vi "Close File.vi"(8 "error in (no error)":errorcluster, 11 "Macro in":refnum<class "Macro.lvclass">) -> (0 "error out":errorcluster, 3 "Macro out":refnum<class "Macro.lvclass">)   [LabVIEW 2020, in "MacroAssert.lvlib" / "Macro.lvclass"]
uses:
  Macro.lvclass
  Macro.lvclass/Macro.ctl
  <vilib>/Utility/config.llb/NI_LVConfig.lvlib
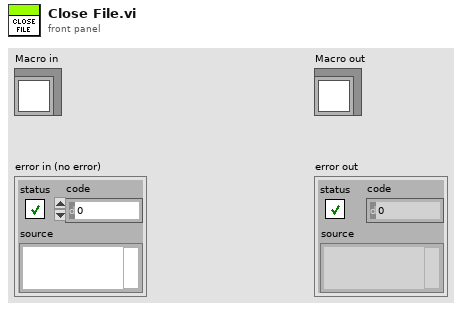
[diagram p1: front panel]
types:
  T1 = typedef "NI_LVConfig.lvlib/Config Data RefNum.ctl" = refnum<k1>
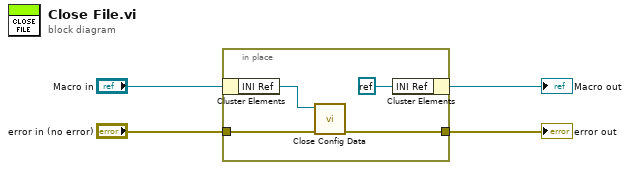
[diagram p0: block diagram]
diagram:
  n1 = in-place {
    in-place-border: "error in (no error)" -> [w8]
    in-place-border: [w7] -> w3
    n2 = in-place-cluster #1("Macro in") -> ("INI Ref"=w5:T1)
    n3 = call <vilib>:"Close Config Data.vi"("error in (no error)"=w8, "refnum"=w5) -> ("error out"=w7:errorcluster)  [unwired: 8 in, 1 out]
    n4 = in-place-cluster #1("INI Ref"=refnum<k0> refnum) -> (→"Macro out":refnum<class "Macro.lvclass">)
  }
  "error out" <- w3
